vi "DistanceComparer.vi"(9 "Data":T1, 10 "Time In":dbl, 11 "Distance In":dbl) -> (3 "Distance Out":dbl)   [LabVIEW 2017]
uses:
  DAQ/Master_DataControl.ctl
  DAQ/TypeDef_cRIOData.ctl
  IMU/TypeDef_IMUData.ctl
  CAN/TypeDef_BMSData.ctl
  CAN/TypeDef_BMS_Status.ctl
  RunTypesLibrary/RunTypeList.ctl
  <vilib>/Analysis/NI_AALPro.lvlib
panel:
  out "Fiducial Sensor Distance":dbl
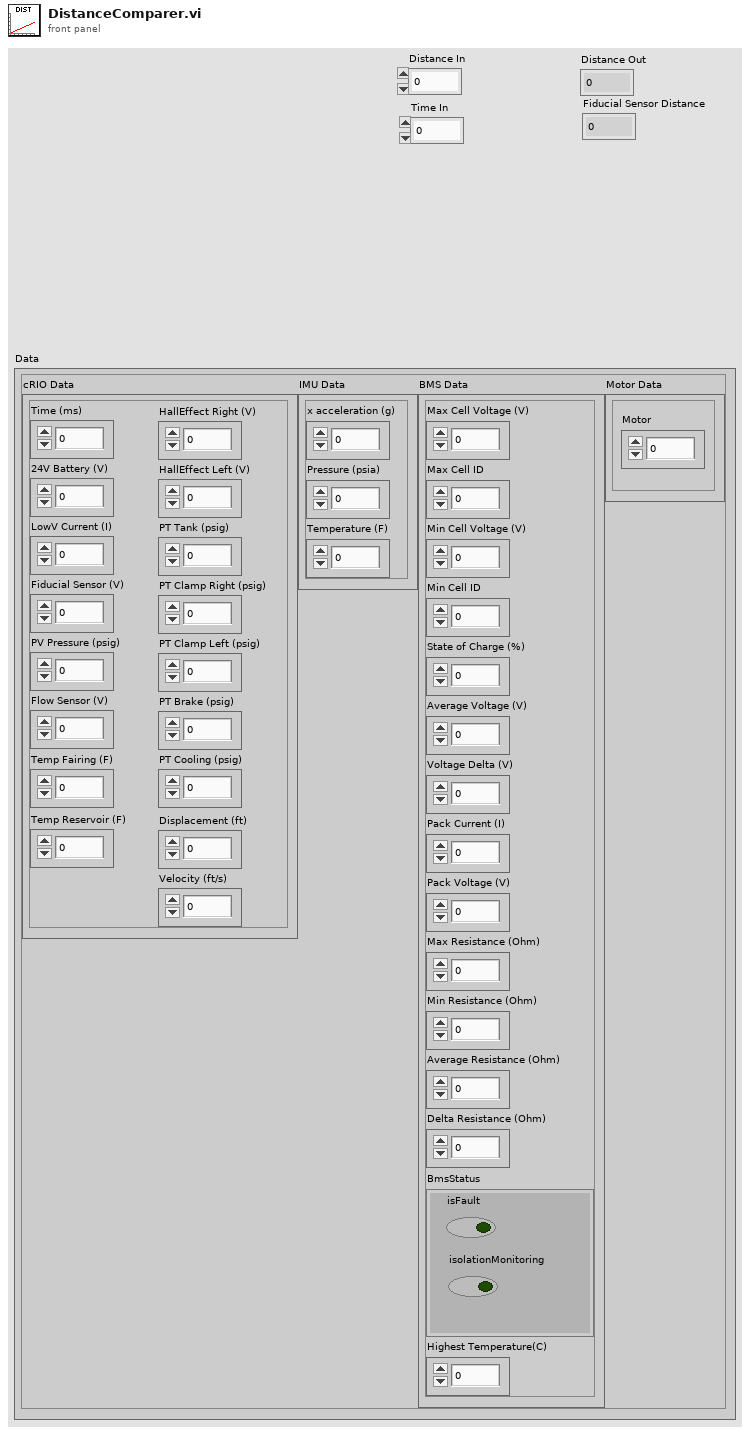
[diagram p1: front panel]
types:
  T1 = typedef "Master_DataControl.ctl" = cluster{"cRIO Data":T2, "IMU Data":T3, "BMS Data":T4, "Motor Data":cluster{"Motor":dbl}}
  T2 = typedef "TypeDef_cRIOData.ctl" = cluster{"Time (ms)":dbl, "24V Battery (V)":dbl, "LowV Current (I)":dbl, "Fiducial Sensor (V)":dbl, "PV Pressure (psig)":dbl, "Flow Sensor (V)":dbl, "Temp Fairing (F)":dbl, "Temp Reservoir (F)":dbl, "HallEffect Right (V)":dbl, "HallEffect Left (V)":dbl, "PT Tank (psig)":dbl, "PT Clamp Right (psig)":dbl, "PT Clamp Left (psig)":dbl, "PT Brake (psig)":dbl, "PT Cooling (psig)":dbl, "Displacement (ft)":dbl, "Velocity (ft/s)":dbl}
  T3 = typedef "TypeDef_IMUData.ctl" = cluster{"x acceleration (g)":dbl, "Pressure (psia)":dbl, "Temperature (F)":dbl}
  T4 = typedef "TypeDef_BMSData.ctl" = cluster{"Max Cell Voltage (V)":dbl, "Max Cell ID":dbl, "Min Cell Voltage (V)":dbl, "Min Cell ID":dbl, "State of Charge (%)":dbl, "Average Voltage (V)":dbl, "Voltage Delta (V)":dbl, "Pack Current (I)":dbl, "Pack Voltage (V)":dbl, "Max Resistance (Ohm)":dbl, "Min Resistance (Ohm)":dbl, "Average Resistance (Ohm)":dbl, "Delta Resistance (Ohm)":dbl, "BmsStatus":T5, "Highest Temperature(C)":dbl}
  T5 = typedef "TypeDef_BMS_Status.ctl" = cluster{"isFault":bool, "isolationMonitoring":bool}
  T6 = typedef "RunTypeList.ctl" = enum16{"Full Run", "Systems Check", "Service"}
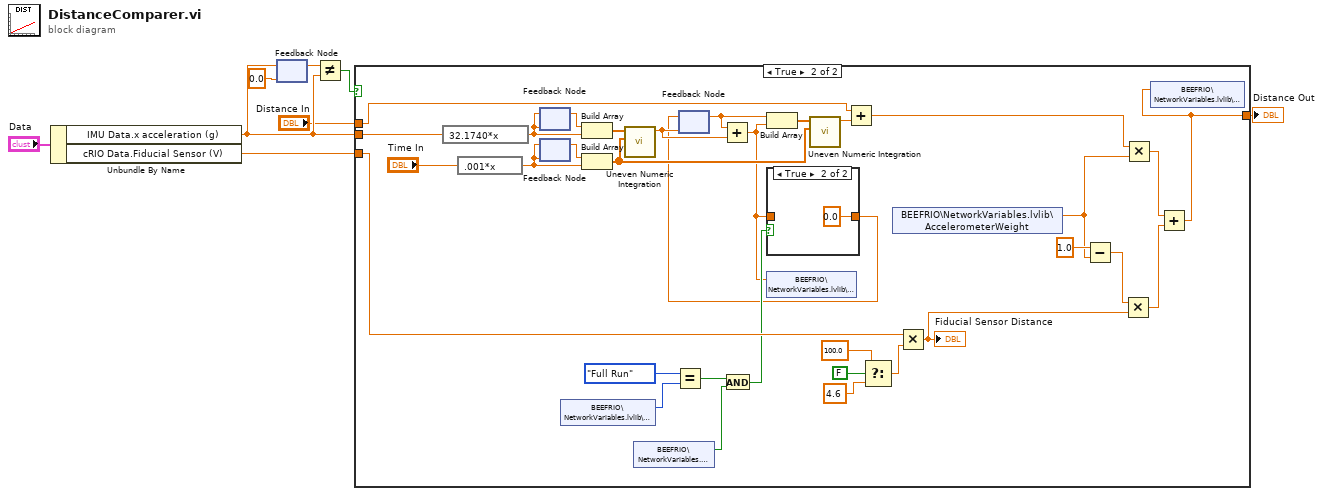
[diagram p0: block diagram]
diagram:
  n1 = Unbundle By Name("Data") -> ("IMU Data.x acceleration (g)"=w5:dbl, "cRIO Data.Fiducial Sensor (V)"=w7:dbl)
  n2 = feedback-in #1(w5) -> ()
  n3 = feedback #1(0.0 ("x acceleration (g)")) -> (w4:dbl)
  n4 = Not Equal?(x=w4, y=w5) -> (x != y?=w3:bool)
  n5 = case shown="True" w3 {
    tunnel: w7 -> [_ w32]
    tunnel: w5 -> [_ w31]
    tunnel: "Distance In" -> [w9 w30]
    tunnel: [w9 w10] -> w1
    frame False {
    }
    frame True {
      n6 = expression code="32.1740*x"(w31) -> (w36:dbl)
      n7 = expression code=".001*x"("Time In") -> (w35:dbl)
      n8 = feedback #2(w36) -> (w37:dbl)
      n9 = feedback-in #2(w36) -> ()
      n10 = feedback #3(w35) -> (w41:dbl)
      n11 = feedback-in #3(w35) -> ()
      n12 = shared-variable "BEEFRIO\\NetworkVariables.lvlib\\RunType"() -> (w28:T6)  [unwired: 1 in, 1 out]
      n13 = Build Array(w37, w36) -> (w40:dbl[])
      n14 = Build Array(w41, w35) -> (w38:dbl[])
      n15 = call <vilib>:"Uneven Numeric Integration.vi"("T"=w38, "X"=w40) -> ("result"=w34:dbl)  [unwired: 8 in, 1 out]
      n16 = shared-variable "BEEFRIO\\NetworkVariables.lvlib\\Ready"() -> (w25:bool)  [unwired: 1 in, 1 out]
      n17 = Equal?(x=RunTypeList."Full Run", y=w28) -> (x = y?=w26:bool)
      n18 = feedback #4(w34) -> (w29:dbl)
      n19 = Add(x=w29, y=w34) -> (x+y=w23:dbl)
      n20 = And(x=w26, y=w25) -> (x .and. y?=w24:bool)
      n21 = Build Array(w29, w23) -> (w39:dbl[])
      n22 = case shown="True" w24 {
        tunnel: w23 -> [w43 _]
        tunnel: [w43 0.0] -> w22
        frame False {
        }
        frame True {
        }
      }
      n23 = feedback-in #4(w22) -> ()
      n24 = shared-variable "BEEFRIO\\NetworkVariables.lvlib\\Velocity"(w23) -> ()  [unwired: 1 in, 1 out]
      n25 = call <vilib>:"Uneven Numeric Integration.vi"("T"=w38, "X"=w39) -> ("result"=w33:dbl)  [unwired: 8 in, 1 out]
      n26 = Add(x=w30, y=w33) -> (x+y=w13:dbl)
      n27 = Select(t=100.0 ("y"), s=FALSE, f=4.6 ("y")) -> (s? t:f=w19:dbl)
      n28 = shared-variable "BEEFRIO\\NetworkVariables.lvlib\\AccelerometerWeight"() -> (w14:sgl)  [unwired: 1 in, 1 out]
      n29 = Multiply(x=w32, y=w19) -> (x*y=w15:dbl)
      "Fiducial Sensor Distance" <- w15
      n30 = Subtract(x=1.0, y=w14) -> (x-y=w16:dbl)
      n31 = Multiply(x=w16, y=w15) -> (x*y=w12:dbl)
      n32 = Multiply(x=w13, y=w14) -> (x*y=w11:dbl)
      n33 = Add(x=w11, y=w12) -> (x+y=w10:dbl)
      n34 = shared-variable "BEEFRIO\\NetworkVariables.lvlib\\Distance"(w10) -> ()  [unwired: 1 in, 1 out]
    }
  }
  "Distance Out" <- w1
